vi "Th2829NX_INIT.vi"(11 "VISA资源名称输出":refnum<visa-resource-name>) -> (3 "VISA资源名称输出 2":refnum<visa-resource-name>)   [LabVIEW 2018]
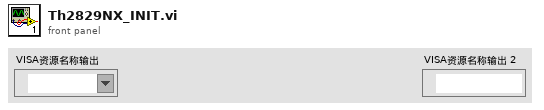
[diagram p1: front panel]
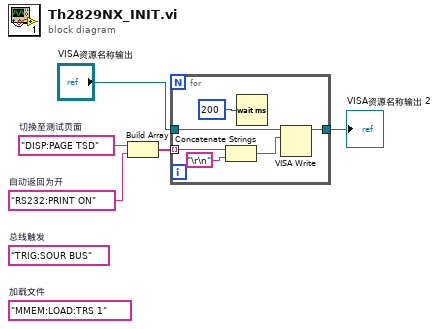
[diagram p0: block diagram]
diagram:
  (unwired) "MMEM:LOAD:TRS 1"  # 加载文件
  (unwired) "TRIG:SOUR BUS"  # 总线触发
  w4 = "RS232:PRINT ON"  # 自动返回为开
  w5 = "DISP:PAGE TSD"  # 切换至测试页面
  n1 = Build Array(w5, w4) -> (w3:string[])
  n2 = for {
    tunnel: w3 -> [w8] mode=indexing
    tunnel: "VISA资源名称输出" -> [w11]
    tunnel: [w9] -> w2
    n3 = Concatenate Strings(w8, "\r\n") -> (w7:string)
    n4 = Wait (ms)(milliseconds to wait=u32 200 ("等待时间（毫秒）")) -> ()  [unwired: 1 out]
    n5 = VISA Write(VISA resource name=w11, write buffer=w7) -> (VISA resource name out=w9:refnum<visa-resource-name>)  [unwired: 1 in, 2 out]
  }
  "VISA资源名称输出 2" <- w2
